vi "Find All Hardware Custom Devices.vi"(8 "error in (no error)":errorcluster, 11 "Routing and Faulting Ref in":T1 format="%.0x") -> (0 "error out":errorcluster, 2 "Hardware Refs":T1[](array[typedef]) format="%.0x", 3 "Routing and Faulting Ref out":T1 format="%.0x")   [LabVIEW 2017, in "Routing and Faulting Hardware API.lvlib"]
uses:
  Routing and Faulting Hardware API.lvlib
  <vilib>/NI Veristand/Custom Device API/Custom Device Item Ref.ctl
  Routing and Faulting/Shared/Constants.vi
  <vilib>/NI Veristand/Custom Device API/Custom Device API.lvlib
  Routing and Faulting/Shared/Routing and Faulting Shared.lvlib
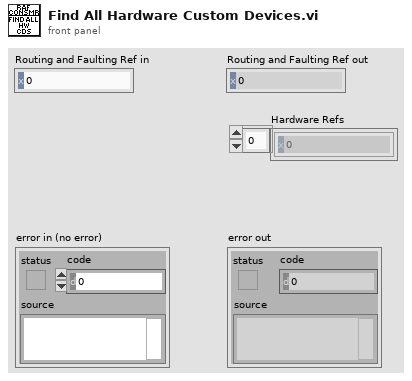
[diagram p1: front panel]
types:
  T1 = typedef "Custom Device API.lvlib/Custom Device Item Ref.ctl" = u64
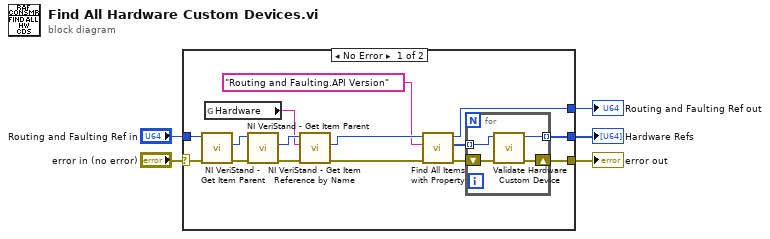
[diagram p0: block diagram]
diagram:
  n1 = case shown="No Error" "error in (no error)" {
    selector: "error in (no error)" -> [w12 w26]
    tunnel: [w20 w26] -> w4
    tunnel: "Routing and Faulting Ref in" -> [w10 w25]
    tunnel: [w19 w25] -> w2
    tunnel: [w18 _] -> w1
    frame No Error {
      n2 = call <vilib>:"NI VeriStand - Get Item Parent.vi"("error in (no error)"=w12, "Item Ref in"=w10) -> ("error out"=w17:errorcluster, "Parent Ref"=w16:T1)  [unwired: 6 in, 2 out]
      n3 = global read "Constants.vi" "Hardware"() -> (w13:string)
      n4 = call <vilib>:"NI VeriStand - Get Item Parent.vi"("error in (no error)"=w17, "Item Ref in"=w16) -> ("error out"=w14:errorcluster, "Parent Ref"=w15:T1)  [unwired: 6 in, 2 out]
      n5 = call <vilib>:"NI VeriStand - Get Item Reference by Name.vi"("error in (no error)"=w14, "Item Name"=w13, "Parent Ref in"=w15) -> ("error out"=w11:errorcluster, "Item Ref"=w9:T1)  [unwired: 5 in, 2 out]
      n6 = call "Find All Items with Property.vi"("error in"=w11, "Property Name"="Routing and Faulting.API Version", "Section Ref in"=w9) -> ("error out"=w7:errorcluster, "Item Refs"=w6:T1[], "Section Ref out"=w19:T1)  [unwired: 5 in, 1 out]
      n7 = for {
        shift-right: [w22] -> w20
        shift-left: w7 -> [w21]
        tunnel: [w24] -> w18 mode=indexing
        tunnel: w6 -> [w23] mode=indexing
        n8 = call "Validate Hardware Custom Device.vi"("error in (no error)"=w21, "Hardware Ref in"=w23) -> ("error out"=w22:errorcluster, "Hardware Ref out"=w24:T1)  [unwired: 8 in]
      }
    }
    frame Error {
    }
  }
  "Routing and Faulting Ref out" <- w2
  "error out" <- w4
  "Hardware Refs" <- w1
